vi "UnblockWait2.vi"(1 "TimeLimit(ms)":u16, 2 "Function":enum16{"Initial", "Timeout?"}(ring), 3 "Name":string) -> (0 "IsTimeout":bool)   [LabVIEW 2016]
panel:
  in  "WaitEntries":T1(array[cluster])
  out "Running":bool
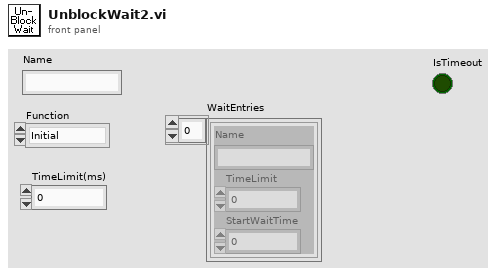
[diagram p1: front panel]
types:
  T1 = cluster{"Name":string, "TimeLimit":u32, "StartWaitTime":u32}[]
  T2 = cluster{"Name":string, "TimeLimit":u32, "StartWaitTime":u32}
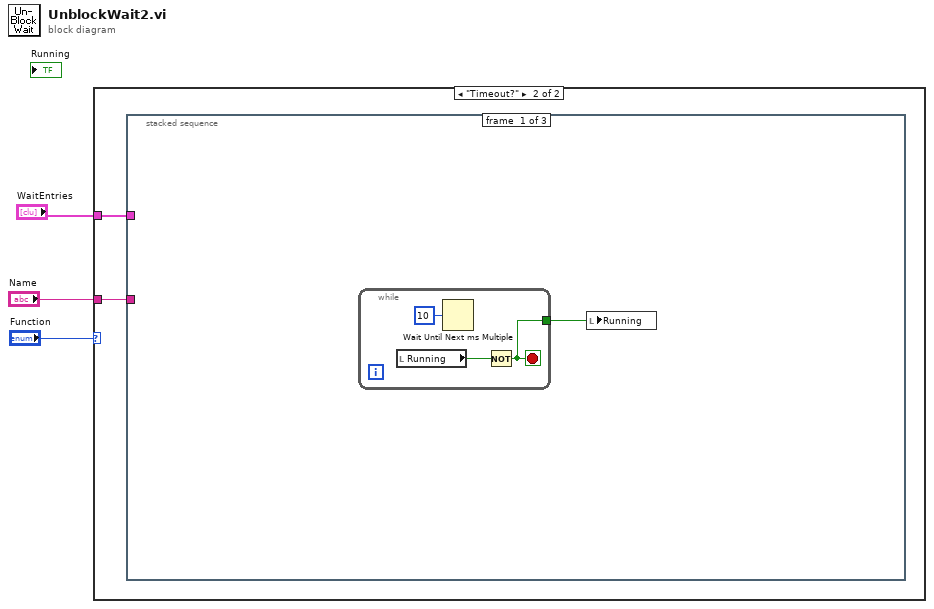
[diagram p0: block diagram]
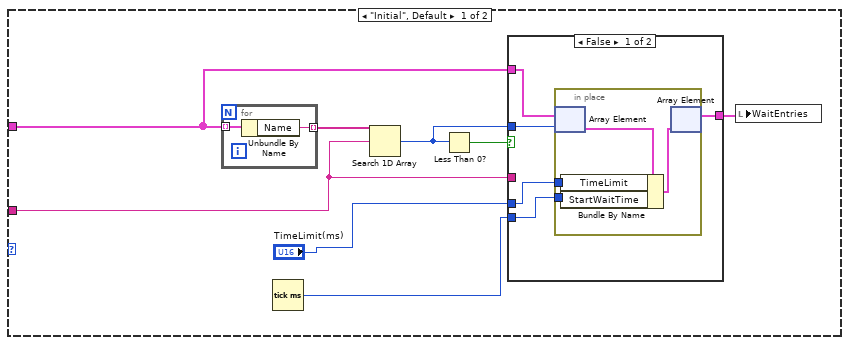
[diagram p2: hidden frame]
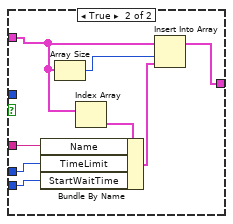
[diagram p3: hidden frame]
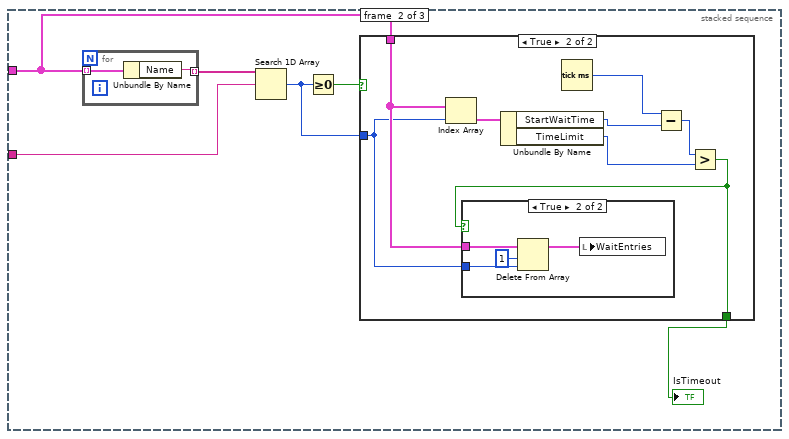
[diagram p4: hidden frame]
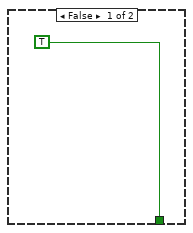
[diagram p5: hidden frame]
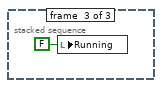
[diagram p7: hidden frame]
diagram:
  n1 = case shown="\"Timeout?\"" "Function" {
    tunnel: "Name" -> [w8 w31]
    tunnel: "WaitEntries" -> [w4 w32]
    frame "Initial", Default {
      n2 = for {
        tunnel: w4 -> [w30] mode=indexing
        tunnel: [w29] -> w11 mode=indexing
        n3 = Unbundle By Name(w30) -> ("Name"=w29:string)
      }
      n4 = Tick Count (ms)() -> (millisecond timer value=w6:u32)
      n5 = Search 1D Array(1D array=w11, element=w8) -> (index of element=w9:i32)  [unwired: 1 in]
      n6 = Less Than 0?(x=w9) -> (x < 0?=w10:bool)
      n7 = case shown="False" w10 {
        tunnel: w4 -> [w16 w27]
        tunnel: w9 -> [w15 _]
        tunnel: w8 -> [_ w25]
        tunnel: "TimeLimit(ms)" -> [w14 w24]
        tunnel: w6 -> [w13 w23]
        tunnel: [w12 w21] -> w5
        frame False {
          n8 = in-place {
            in-place-border: w14 -> [w18]
            in-place-border: w13 -> [w17]
            n9 = in-place-array #1(w16, w15) -> (w20:T2)
            n10 = Bundle By Name(cluster=w20, "TimeLimit"=w18, "StartWaitTime"=w17) -> (w19:T2)
            n11 = in-place-array #1(w19) -> (w12:T1)  [unwired: 1 out]
          }
        }
        frame True {
          n12 = Array Size(array=w27) -> (size(s)=w28:i32)
          n13 = Index Array(array=w27) -> (element=w26:T2)  [unwired: 1 in]
          n14 = Bundle By Name(cluster=w26, "Name"=w25, "TimeLimit"=w24, "StartWaitTime"=w23) -> (w22:T2)
          n15 = Insert Into Array(array=w27, index=w28, new element=w22) -> (w21:T1)
        }
      }
      n16 = local write "WaitEntries"(w5) -> ()
    }
    frame "Timeout?" {
      n17 = stacked-sequence {
        tunnel: w32 -> [_ w38 _]
        tunnel: w31 -> [_ w41 _]
        frame #0 {
          n18 = while {
            tunnel: [w34] -> w33
            stop <- w34 stop-if-true
            n19 = local read "Running"() -> (w36:bool)
            n20 = Wait Until Next ms Multiple(millisecond multiple=u32 10) -> ()  [unwired: 1 out]
            n21 = Not(x=w36) -> (.not. x?=w34:bool)
          }
          n22 = local write "Running"(w33) -> ()
        }
        frame #1 {
          n23 = for {
            tunnel: w38 -> [w57] mode=indexing
            tunnel: [w56] -> w42 mode=indexing
            n24 = Unbundle By Name(w57) -> ("Name"=w56:string)
          }
          n25 = Search 1D Array(1D array=w42, element=w41) -> (index of element=w39:i32)  [unwired: 1 in]
          n26 = Greater Or Equal To 0?(x=w39) -> (x >= 0?=w40:bool)
          n27 = case shown="True" w40 {
            tunnel: w39 -> [_ w45]
            tunnel: w38 -> [_ w46]
            tunnel: [TRUE w44] -> w37
            frame False {
            }
            frame True {
              n28 = Index Array(array=w46, index=w45) -> (element=w51:T2)
              n29 = Unbundle By Name(w51) -> ("StartWaitTime"=w49:u32, "TimeLimit"=w47:u32)
              n30 = Tick Count (ms)() -> (millisecond timer value=w50:u32)
              n31 = Subtract(x=w50, y=w49) -> (x-y=w48:u32)
              n32 = Greater?(x=w48, y=w47) -> (0:w44:bool)
              n33 = case shown="True" w44 {
                tunnel: w46 -> [_ w55]
                tunnel: w45 -> [_ w54]
                frame False {
                }
                frame True {
                  n34 = Delete From Array(array=w55, length=1, index=w54) -> (array with subset deleted=w52:T1)  [unwired: 1 out]
                  n35 = local write "WaitEntries"(w52) -> ()
                }
              }
            }
          }
          "IsTimeout" <- w37
        }
        frame #2 {
          n36 = local write "Running"(FALSE ("Running")) -> ()
        }
      }
    }
  }
